vi "R1DOControl.vi"(8 "error constant":errorcluster, 11 "LabVIEW Web Service":refnum<class "Web Service.lvclass">) -> ()   [LabVIEW 2016]
uses:
  <vilib>/wsapi/Web Service.lvclass
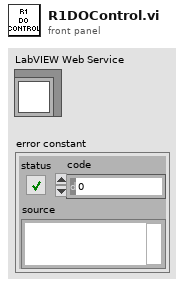
[diagram p1: front panel]
types:
  T1 = cluster{"Media Pump":bool, "Water Pump":bool, "Effluent Pump":bool, "Release Valve":bool, "Gas Pump":bool}
  T2 = cluster{"Set Point, mg/L":dbl, "Tolerance, mg/L":dbl, "N2 Valve Gain":dbl, "Air Valve Gain":dbl}
  T3 = cluster{"Signal, mA":dbl, "Value, UNITS HERE":dbl}
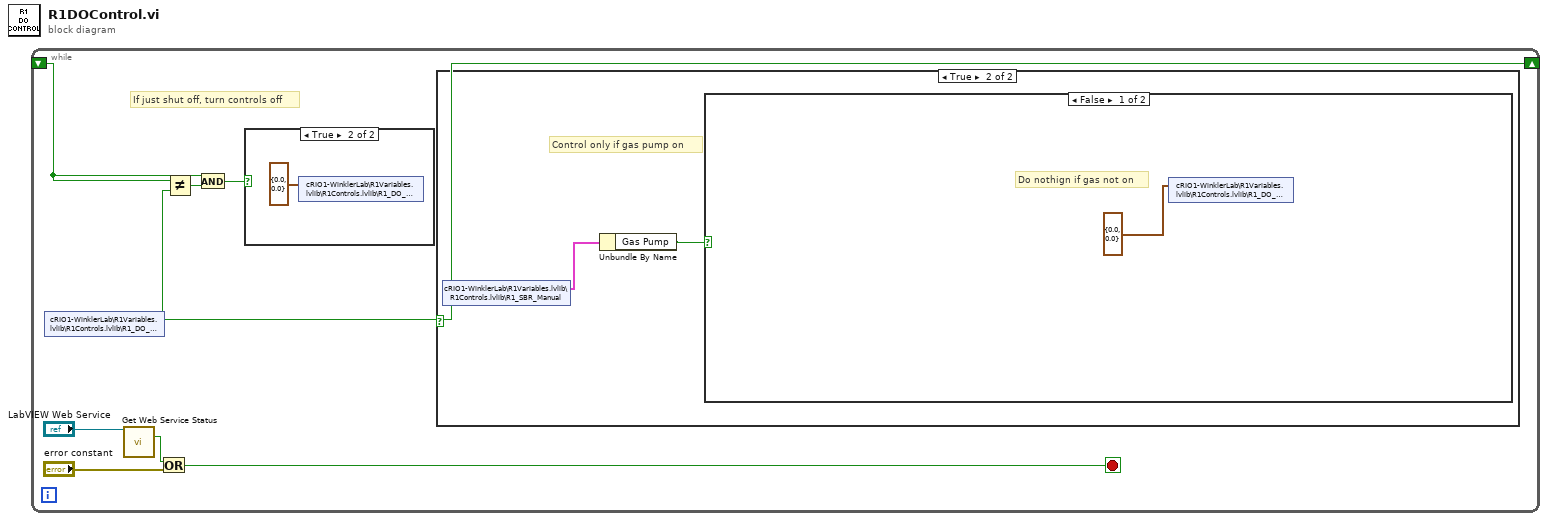
[diagram p0: block diagram]
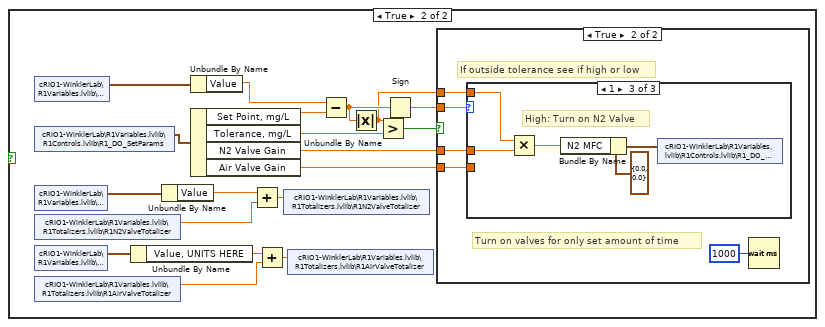
[diagram p4: hidden frame]
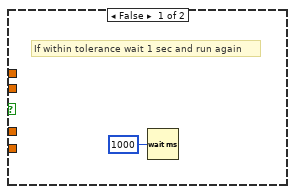
[diagram p5: hidden frame]
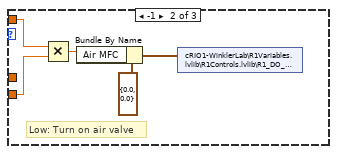
[diagram p7: hidden frame]
diagram:
  n1 = while {
    shift-right: [w3] -> _
    shift-left: _ -> [w1]
    stop <- w5 stop-if-true
    # "If just shut off, turn controls off"
    n2 = shared-variable "cRIO1-WinklerLab\\R1Variables.lvlib\\R1Controls.lvlib\\R1_DO_Switch"() -> (w3:bool)  [unwired: 1 in, 1 out]
    n3 = call <vilib>:"Get Web Service Status.vi"("LabVIEW Web Service"="LabVIEW Web Service") -> ("service stopping?"=w8:bool)  [unwired: 12 in, 2 out]
    n4 = Or(x=w8, y="error constant") -> (x .or. y?=w5:bool)
    n5 = Not Equal?(x=w1, y=w3) -> (x != y?=w2:bool)
    n6 = And(x=w1, y=w2) -> (x .and. y?=w4:bool)
    n7 = case shown="True" w4 {
      frame False {
      }
      frame True {
        n8 = shared-variable "cRIO1-WinklerLab\\R1Variables.lvlib\\R1Controls.lvlib\\R1_DO_Manual"(cluster{"Air MFC":dbl, "N2 MFC":dbl} {"Air MFC"=0.0, "N2 MFC"=0.0} ("R1DOManual")) -> ()  [unwired: 1 in, 1 out]
      }
    }
    n9 = case shown="True" w3 {
      frame False {
        # "Don't do anything if control is off"
      }
      frame True {
        # "Control only if gas pump on"
        n10 = shared-variable "cRIO1-WinklerLab\\R1Variables.lvlib\\R1Controls.lvlib\\R1_SBR_Manual"() -> (w10:T1)  [unwired: 1 in, 1 out]
        n11 = Unbundle By Name(w10) -> ("Gas Pump"=w11:bool)
        n12 = case shown="False" w11 {
          frame False {
            # "Do nothign if gas not on"
            n13 = shared-variable "cRIO1-WinklerLab\\R1Variables.lvlib\\R1Controls.lvlib\\R1_DO_Manual"(cluster{"Air MFC":dbl, "N2 MFC":dbl} {"Air MFC"=0.0, "N2 MFC"=0.0} ("R1DOManual")) -> ()  [unwired: 1 in, 1 out]
          }
          frame True {
            n14 = shared-variable "cRIO1-WinklerLab\\R1Variables.lvlib\\R1Signals.lvlib\\R1DO"() -> (w25:cluster{"Signal":dbl, "Value":dbl})  [unwired: 1 in, 1 out]
            n15 = shared-variable "cRIO1-WinklerLab\\R1Variables.lvlib\\R1Controls.lvlib\\R1_DO_SetParams"() -> (w24:T2)  [unwired: 1 in, 1 out]
            n16 = shared-variable "cRIO1-WinklerLab\\R1Variables.lvlib\\R1Signals.lvlib\\R1N2"() -> (w20:cluster{"Signal":dbl, "Value":dbl})  [unwired: 1 in, 1 out]
            n17 = shared-variable "cRIO1-WinklerLab\\R1Variables.lvlib\\R1Totalizers.lvlib\\R1N2ValveTotalizer"() -> (w14:dbl)  [unwired: 1 in, 1 out]
            n18 = shared-variable "cRIO1-WinklerLab\\R1Variables.lvlib\\R1Signals.lvlib\\R1Air"() -> (w19:T3)  [unwired: 1 in, 1 out]
            n19 = shared-variable "cRIO1-WinklerLab\\R1Variables.lvlib\\R1Totalizers.lvlib\\R1AirValveTotalizer"() -> (w17:dbl)  [unwired: 1 in, 1 out]
            n20 = Unbundle By Name(w19) -> ("Value, UNITS HERE"=w18:dbl)
            n21 = Unbundle By Name(w20) -> ("Value"=w15:dbl)
            n22 = Unbundle By Name(w25) -> ("Value"=w31:dbl)
            n23 = Unbundle By Name(w24) -> ("Set Point, mg/L"=w30:dbl, "Tolerance, mg/L"=w29:dbl, "N2 Valve Gain"=w26:dbl, "Air Valve Gain"=w23:dbl)
            n24 = Add(x=w15, y=w14) -> (x+y=w13:dbl)
            n25 = Add(x=w18, y=w17) -> (x+y=w16:dbl)
            n26 = shared-variable "cRIO1-WinklerLab\\R1Variables.lvlib\\R1Totalizers.lvlib\\R1N2ValveTotalizer"(w13) -> ()  [unwired: 1 in, 1 out]
            n27 = shared-variable "cRIO1-WinklerLab\\R1Variables.lvlib\\R1Totalizers.lvlib\\R1AirValveTotalizer"(w16) -> ()  [unwired: 1 in, 1 out]
            n28 = Subtract(x=w31, y=w30) -> (x-y=w22:dbl)
            n29 = Absolute Value(x=w22) -> (abs(x)=w21:dbl)
            n30 = Greater?(x=w21, y=w29) -> (0:w28:bool)
            n31 = Sign(1:w22) -> (0:w27:dbl)
            n32 = case shown="True" w28 {
              tunnel: w27 -> [_ w37]
              tunnel: w26 -> [_ w36]
              tunnel: w23 -> [_ w35]
              tunnel: w21 -> [_ w34]
              frame False {
                # "If within tolerance wait 1 sec and run again"
                n33 = Wait (ms)(milliseconds to wait=u32 1000) -> ()  [unwired: 1 out]
              }
              frame True {
                # "Turn on valves for only set amount of time"
                # "If outside tolerance see if high or low"
                n34 = case shown="1" w37 {
                  tunnel: w35 -> [_ w39 _]
                  tunnel: w36 -> [_ _ w45]
                  tunnel: w34 -> [_ w40 w46]
                  frame 0, Default {
                    # "Unless tolerance is 0 this code\nshouldn't be accesible"
                  }
                  frame -1 {
                    # "Low: Turn on air valve"
                    n35 = Multiply(x=w40, y=w39) -> (x*y=w41:dbl)
                    n36 = Bundle By Name(cluster=cluster{"Air MFC":dbl, "N2 MFC":dbl} {"Air MFC"=0.0, "N2 MFC"=0.0} ("R1DOManual"), "Air MFC"=w41) -> (w38:cluster{"Air MFC":dbl, "N2 MFC":dbl})
                    n37 = shared-variable "cRIO1-WinklerLab\\R1Variables.lvlib\\R1Controls.lvlib\\R1_DO_Manual"(w38) -> ()  [unwired: 1 in, 1 out]
                  }
                  frame 1 {
                    # "High: Turn on N2 Valve"
                    n38 = Multiply(x=w46, y=w45) -> (x*y=w44:dbl)
                    n39 = Bundle By Name(cluster=cluster{"Air MFC":dbl, "N2 MFC":dbl} {"Air MFC"=0.0, "N2 MFC"=0.0} ("R1DOManual"), "N2 MFC"=w44) -> (w43:cluster{"Air MFC":dbl, "N2 MFC":dbl})
                    n40 = shared-variable "cRIO1-WinklerLab\\R1Variables.lvlib\\R1Controls.lvlib\\R1_DO_Manual"(w43) -> ()  [unwired: 1 in, 1 out]
                  }
                }
                n41 = Wait (ms)(milliseconds to wait=u32 1000) -> ()  [unwired: 1 out]
              }
            }
          }
        }
      }
    }
  }
